vi "build_settings_pck.vi"(8 "value":u16, 11 "SETTINGS_Cmd":T1) -> (3 "SETTINGS_Pck":T2)   [LabVIEW 2021]
uses:
  typedefs/SETTINGS_Pck.ctl
  typedefs/SETTINGS_Cmd.ctl
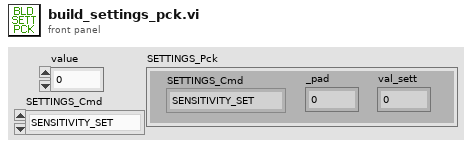
[diagram p1: front panel]
types:
  T1 = typedef "SETTINGS_Cmd.ctl" = enum8{"SENSITIVITY_SET", "SENSITIVITY_VAL", "RECORD_TIME_SET", "RECORD_TIME_VAL", "DISC_FREQ_SET", "DISC_FREQ_VAL", "STATE_SET", "STATE_VAL"}
  T2 = typedef "SETTINGS_Pck.ctl" = cluster{"SETTINGS_Cmd":T1, "_pad":u8, "val_sett":u16}
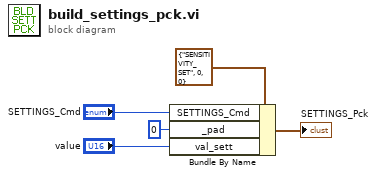
[diagram p0: block diagram]
diagram:
  n1 = Bundle By Name(cluster=T2 {"SETTINGS_Cmd"=enum."SENSITIVITY_SET", "_pad"=0, "val_sett"=0} ("SETTINGS_Pck"), "SETTINGS_Cmd"="SETTINGS_Cmd", "_pad"=u8 0, "val_sett"="value") -> (→"SETTINGS_Pck":T2)
